vi "calcActForce.vi"(8 "error in (no error)":errorcluster, 9 "Mirror DOF (um)":dbl[](array[numeric]), 10 "Mirror":enum16{"M1M3", "M2"}(ring), 11 "BendModeToForce in":refnum<class "BendModeToForce.lvclass">) -> (0 "error out":errorcluster, 2 "Actuator Force (N)":dbl[](array[numeric]), 3 "BendModeToForce out":refnum<class "BendModeToForce.lvclass">)   [LabVIEW 2016, in "BendModeToForce.lvclass"]
doc: "Calculate the actuator forces in N based on the mirror type and degree of freedom (DOF) in um."
uses:
  BendModeToForce.lvclass
  BendModeToForce.lvclass/BendModeToForce.ctl
  <vilib>/Analysis/baseanly.llb/Real A x B.vi
  <vilib>/Analysis/Matrix/Numeric/Conversions/Array To Matrix - RA.vi
  <vilib>/Analysis/Matrix/Numeric/Conversions/Array To Matrix - RA2.vi
  <vilib>/Analysis/Matrix/Numeric/Conversions/Matrix To Array - RM.vi
  <vilib>/Analysis/Matrix/NI_Matrix.lvlib
  <vilib>/Analysis/NI_AALBase.lvlib
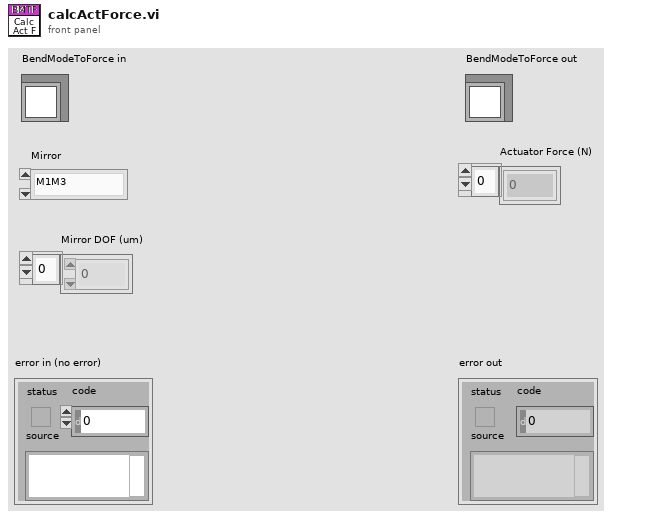
[diagram p1: front panel]
types:
  T1 = typedef "NI_Matrix.lvlib/RealMatrix.ctl" = dbl[][]
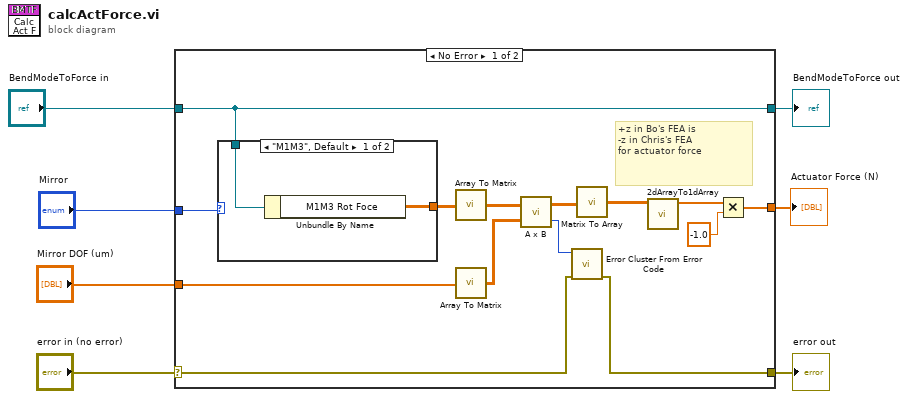
[diagram p0: block diagram]
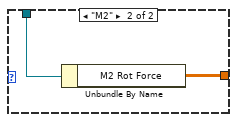
[diagram p2: hidden frame]
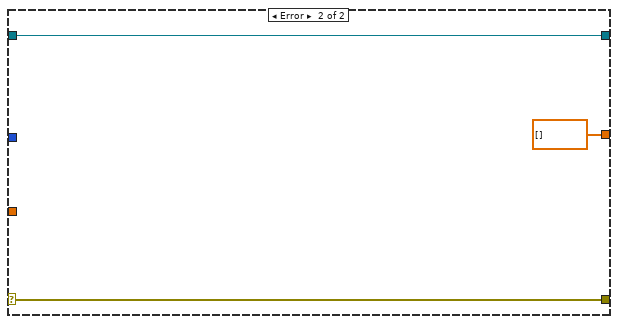
[diagram p3: hidden frame]
diagram:
  n1 = case shown="No Error" "error in (no error)" {
    selector: "error in (no error)" -> [w14 w28]
    tunnel: [w13 w28] -> w6
    tunnel: [w20 w27] -> w4
    tunnel: "BendModeToForce in" -> [w20 w27]
    tunnel: "Mirror" -> [w21 _]
    tunnel: "Mirror DOF (um)" -> [w18 _]
    tunnel: [w10 dbl[] [] ("1D Array")] -> w1
    frame No Error {
      # "+z in Bo's FEA is \n-z in Chris's FEA\nfor actuator force"
      n2 = case shown="\"M1M3\", Default" w21 {
        tunnel: w20 -> [w23 w25]
        tunnel: [w22 w24] -> w19
        frame "M1M3", Default {
          n3 = Unbundle By Name(w23) -> ("M1M3 Rot Foce"=w22:dbl[][])
        }
        frame "M2" {
          n4 = Unbundle By Name(w25) -> ("M2 Rot Force"=w24:dbl[][])
        }
      }
      n5 = call-poly <vilib>:"Array To Matrix.vi"("Real 2D Array"=w19) -> ("Real Matrix"=w17:T1)
      n6 = call-poly <vilib>:"Array To Matrix.vi"("Real 1D Array"=w18) -> ("Real Matrix (Column Vector)"=w16:T1)
      n7 = call-poly <vilib>:"A x B.vi"("B"=w16, "A"=w17) -> ("error"=w15:i32, "A x B"=w12:T1)
      n8 = call <vilib>:"Error Cluster From Error Code.vi"("error in (no error)"=w14, "error code (0)"=w15) -> ("error out"=w13:errorcluster)  [unwired: 7 in]
      n9 = call-poly <vilib>:"Matrix To Array.vi"("Real Matrix"=w12) -> ("Real 2D Array"=w11:dbl[][])
      n10 = call "2dArrayTo1dArray.vi"("2D Array"=w11) -> ("1D Array"=w9:dbl[])  [unwired: 10 in]
      n11 = Multiply(x=w9, y=-1.0 ("Numeric")) -> (x*y=w10:dbl[])
    }
    frame Error {
    }
  }
  "error out" <- w6
  "BendModeToForce out" <- w4
  "Actuator Force (N)" <- w1
